vi "tearDown.vi"(8 "error in (no error)":errorcluster, 10 "connection ID":refnum<k5>, 11 "session":T1) -> (0 "error out":errorcluster)   [LabVIEW 2013, in "support.lvlib"]
doc: "Close the session, terminate the connection, and release the library."
uses:
  libssh2/Session Refnum.ctl
  support.lvlib
  libssh2/libssh2.lvlib
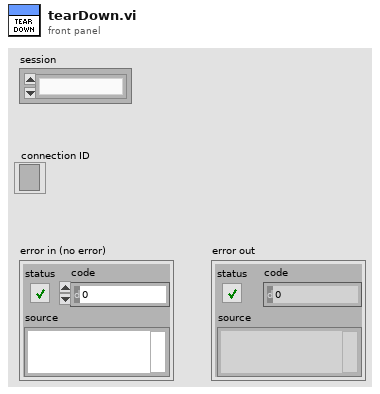
[diagram p1: front panel]
types:
  T1 = typedef "libssh2.lvlib/Session Refnum.ctl" = refnum<k1>
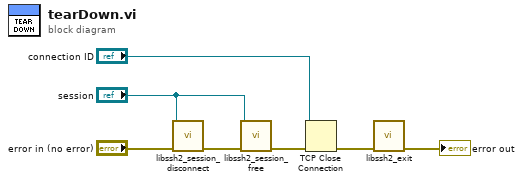
[diagram p0: block diagram]
diagram:
  n1 = call "libssh2_session_disconnect.vi"("error in (no error)"="error in (no error)", "session"="session") -> ("error out"=w5:errorcluster)  [unwired: 9 in]
  n2 = call "libssh2_session_free.vi"("error in (no error)"=w5, "session"="session") -> ("error out"=w7:errorcluster)  [unwired: 9 in]
  n3 = TCP Close Connection(connection ID="connection ID", error in (no error)=w7) -> (error out=w6:errorcluster)  [unwired: 1 in, 1 out]
  n4 = call "libssh2_exit.vi"("error in (no error)"=w6) -> ("error out"=→"error out":errorcluster)  [unwired: 10 in]
